vi "Get Time.vi"(8 "error in (no error)":errorcluster, 11 "BehaviorData in":refnum<class "BehaviorData.lvclass">) -> (0 "error out":errorcluster, 2 "Counter Time":dbl, 3 "BehaviorData out":refnum<class "BehaviorData.lvclass">)   [LabVIEW 2014, in "BehaviorData.lvclass"]
uses:
  BehaviorData.lvclass
  BehaviorData.lvclass/BehaviorData.ctl
  <vilib>/DAQmx/read.llb/DAQmx Read (Counter U32 1Chan 1Samp).vi
panel:
  out "Err":dbl
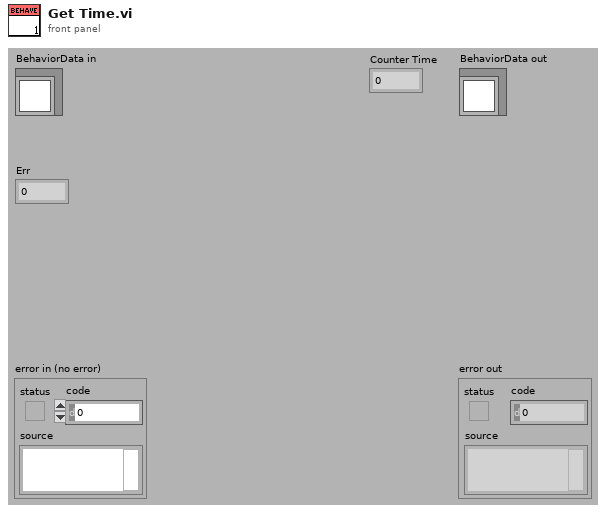
[diagram p1: front panel]
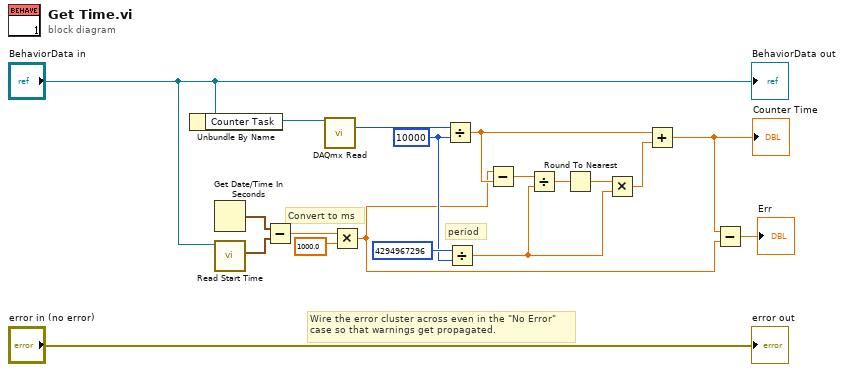
[diagram p0: block diagram]
diagram:
  w12 = u32 10000 ("y")
  # "Convert to ms"
  # "period"
  # "Wire the error cluster across even in the \"No Error\"\ncase so that warnings get propagated."
  n1 = Unbundle By Name("BehaviorData in") -> ("Counter Task"=w17:refnum<k21>)
  n2 = Get Date/Time In Seconds() -> (seconds since 1Jan1904=w15:timestamp)
  n3 = call-dynamic "Read Start Time.vi"("AcquistionObject in"="BehaviorData in") -> ("Start Time"=w14:timestamp)  [unwired: 8 in, 2 out]
  n4 = Subtract(x=w15, y=w14) -> (x-y=w4:dbl)
  n5 = call-poly <vilib>:"DAQmx Read.vi"("task/channels in"=w17) -> ("data"=w16:u32)  [unwired: 12 in, 2 out]
  n6 = Multiply(x=w4, y=1000.0) -> (x*y=w1:dbl)
  n7 = Divide(x=w16, y=w12) -> (x/y=w2:dbl)
  n8 = Divide(x=u64 4294967296, y=w12) -> (x/y=w7:dbl)
  n9 = Subtract(x=w1, y=w2) -> (x-y=w10:dbl)
  n10 = Divide(x=w10, y=w7) -> (x/y=w9:dbl)
  n11 = Round To Nearest(number=w9) -> (nearest integer value=w8:dbl)
  n12 = Multiply(x=w8, y=w7) -> (x*y=w6:dbl)
  n13 = Add(x=w2, y=w6) -> (x+y=w5:dbl)
  "Counter Time" <- w5
  n14 = Subtract(x=w5, y=w1) -> (x-y=→"Err":dbl)
  "error out" <- "error in (no error)"
  "BehaviorData out" <- "BehaviorData in"
